vi "Snap Splitter to Reference.vi"(8 "error in":errorcluster, 10 "splitter on move":refnum<vi>, 11 "reference splitter":refnum<vi>) -> (0 "error out":errorcluster)   [LabVIEW 2020, in "NI_TDMS File Viewer.lvlib"]
uses:
  <vilib>/Utility/TDMS File Viewer/NI_TDMS File Viewer.lvlib
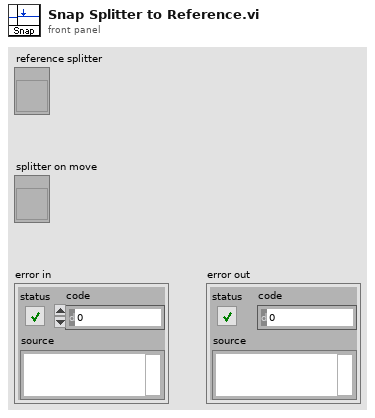
[diagram p1: front panel]
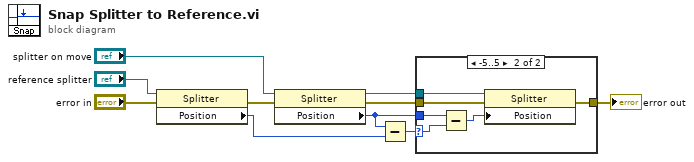
[diagram p0: block diagram]
diagram:
  n1 = property class="Splitter"(reference="reference splitter", error in="error in") -> (error out=w9:errorcluster, "Position"=w4:i32)  [unwired: 1 out]
  n2 = property class="Splitter"(reference="splitter on move", error in=w9) -> (reference out=w3:refnum<vi>, error out=w8:errorcluster, "Position"=w6:i32)
  n3 = Subtract(x=w6, y=w4) -> (x-y=w5:i32)
  n4 = case shown="-5..5" w5 {
    selector: w5 -> [_ w13]
    tunnel: w8 -> [w11 w17]
    tunnel: w3 -> [_ w15]
    tunnel: [w11 w16] -> w10
    tunnel: w6 -> [_ w14]
    frame Default {
    }
    frame -5..5 {
      n5 = Subtract(x=w14, y=w13) -> (x-y=w12:i32)
      n6 = property class="Splitter"(reference=w15, error in=w17, "Position"=w12) -> (error out=w16:errorcluster)  [unwired: 1 out]
    }
  }
  "error out" <- w10
